vi "Solid Dilution Control-5.vi"() -> ()   [LabVIEW 2009]
uses:
  <vilib>/Instr/_visa.llb/VISA Configure Serial Port (Instr).vi
  <vilib>/DAQmx/configure/timing.llb/DAQmx Timing (Sample Clock).vi
  <vilib>/DAQmx/create/channels.llb/DAQmx Create Channel (AI-Strain-Strain Gage).vi
  <vilib>/DAQmx/read.llb/DAQmx Read (Analog 1D DBL 1Chan NSamp).vi
  <vilib>/Analysis/NI_AALBase.lvlib
panel:
  out "Target = Soln Size?":bool=TRUE
  in  "Fill Target":dbl=900.0
  out "Hydration (g)":dbl
  in  "SIM MASS":dbl=900.0
  in  "real":bool=TRUE
  out "# of Rows Saved":i32
  out "DAQ Loop":i32=644
  out "SCB Loop":i32=51
  out "Save Loop":i32=66
  out "Main Loop":i32=645
  out "Event Loop":i32=36
  in  "Tab Control":enum32{"DISPLAY", "CONFIGURE", "Load Cell"}(tab)
  in  "Settings":T1={"ON Settings"={"Enable Dynamic Setpoint?"=TRUE, "Enable Dynamic Dispense Time?"=TRUE, "Enable Drain Rate Functions"=TRUE, "Dispense Sample Time (s)"=0.1, "Mass Average Samples"=20, "ON Timeout (sec)"=300.0, "1st Setpoint (% of Target)"=90.0, "2nd Setpoint (% of Target)"=95.0, "3rd Setpoint (% of Target)"=100.0, "Measure Dispense Delay (sec)"=10.0, "Minimum Spray Time (s)"=2.0}, "OFF Settings"={"Drain Sample Time (s)"=0.1, "Drain Rate Ave Size"=100, "Drain Rate Limits (± g/sec)"=100.0, "Level Slope Range (± g/sec)"=0.05, "OFF Timeout (sec)"=300.0, "Near SP Slope Level (± g/sec)"=0.005, "Near Setpoint Threshold (%)"=99.0}, "Overshoot Settings"={"Time Limit (s)"=30.0, "Container MAX (g)"=1500.0, "Max FILL Slope (+/- g/sec)"=100.0, "% Overshot to Enable (>)"=3.0}, "FILL Timeout (s)"=300.0, "Full \nSettle Time (s)"=30.0, "Pre-Hydrate \nSpray Time (s)"=10.0, "Pre-Hydrate \nWait Time (s)"=30.0} {"OFF Settings"."Near SP Slope Level (± g/sec)" format="%.3g"; "OFF Settings"."Level Slope Range (± g/sec)" format="%.3g"}
  out "Values":T2 {"Drain Time (s)" format="%.2f"; "Drain Rate (g/sec)" format="%.2f"; "Spray Mass Loss (g)" format="%.2f"; "Time Elapsed (s)" format="%.2f"; "Time Target (s)" format="%.2f"; "Dynamic Setpoint (g)" format="%.2f"; "Static Setpoint (g)" format="%.2f"; "Grams to Setpoint" format="%.2f"; "Adjusted Mass (g)" format="%.2f"; "Dispense Rate (g/sec)" format="%.2f"; "Fill Mass (g)" format="%.2f"; "Fill Rate (g/sec)" format="%.2f"}
  in  "Tare":bool
  in  "Settings Button":bool
  in  "START Dispense":bool
  in  "STOP Dispense":bool
  in  "Fill Setpoint (g)":dbl
  in  "Dispense Setpoint (%)":dbl=10.0
  out "Mass Chart":T3(graph)={"Grams (SCB)"=0.0, "Fill Target"=900.0, "Dispense Target"=0.0}
  out "Signals":T4={"Dispense"=FALSE, "Fill"=FALSE, "Spray"=FALSE, "Drain"=TRUE, "Complete"=FALSE, "Fill Error"=FALSE, "Dispense Error"=FALSE, "Fill Timeout"=FALSE, "Dispense Timeout"=FALSE}
  in  "Overshoot Adjust?":bool
  out "Dispense Mode":T5(ring)
  out "Product Mass (g)":dbl format="%.2f"
  in  "Solution Size (g)":dbl=1000.0
  in  "Save Interval (s)":dbl=1.0
  in  "Write/Read Wait (ms)":u32=100
  in  "Event Loop Wait (ms)":i32=5000
  in  "File Path Input":path
  out "SCB Error":errorcluster={"status"=TRUE, "code"=-1073807343, "source"="Property Node (arg 1) in Read SCB via ESP (SubVI).vi->Solid Dilution Control-5.vi"}
  out "SCB Output":T6
  in  "SCB COM Port":refnum<visa-resource-name>="COM5"
  in  "SCB Baud Rate":u32=9600
  in  "DAQ COM Port":refnum<visa-resource-name>="COM4"
  in  "DAQ Baud Rate":u32=115200
  in  "Minimum Wait (ms)":u32=100
  in  "Module Address":i32=1
  in  "Relay Control":T7
  out "DAQ Com Error":errorcluster={"status"=TRUE, "code"=-1073807343, "source"="Property Node (arg 1) in VISA Configure Serial Port (Instr).vi->Solid Dilution Control-5.vi"}
  out "DAQ Error":errorcluster={"status"=TRUE, "code"=-1073807343, "source"="VISA Write in 7067 Relay Module (SubVI).vi->Solid Dilution Control-5.vi"}
  out "Relays Active?":bool
  out "SCB Com Error":errorcluster={"status"=TRUE, "code"=-1073807343, "source"="Property Node (arg 1) in VISA Configure Serial Port (Instr).vi->Solid Dilution Control-5.vi"}
  out "Save Error":errorcluster caption="Error Output"
  out "Weight (Grams)":dbl format="%.2f"
  out "Product Values":T8
  out "Spray Count":i32
  out "CDAQ Array":dbl[](graph)
  out "Grams (Tedea 1040 CDAQ)":dbl[](graph)
  in  "Minimum Value":dbl=-0.001 format="%0.3f"
  in  "Maximum Value":dbl=0.001 format="%0.3f"
  in  "CDAQ Channel":tag="Dev2/ai1"
  out "CDAQ Error":errorcluster={"status"=TRUE, "code"=-200220, "source"="DAQmx Create Channel (AI-Strain-Strain Gage).vi:1<append>\n<B>Device Specified: </B>Dev2\n\n<B>Task Name: </B>_unnamedTask<4>"}
  out "Raw Ave (Tedea 1040 CDAQ)":dbl=nan
  in  "Y LO (g)":dbl
  in  "Y HI (g)":dbl=5000.0
  in  "Set HI":bool
  in  "Set LO":bool
  out "CDAQ Sample Size":i32
  in  "CDAQ Wait (ms)":u32=100
  in  "CDAQ RATE":dbl=1000.0 caption="Rate" format="%0.2f"
  out "CDAQ Loop":i32
  in  "LO":dbl
  in  "HI":dbl
  in  "Save (Enable/Signal)":bool
  in  "STOP PROGRAM":bool
  # "SOLID DILUTION CONTROL SYSTEM"
  # "Program Last Updated 7/13/2010"
  # "SAVE\nENABLE"
  # "Blake Otting - Systems Engineering Lab - 2009 /2010"
  # "DISPENSE CONTROL"
  # "ONLY ADJUST\nBOLD VALUES!"
  # "GRAMS"
  # "SIGNAL"
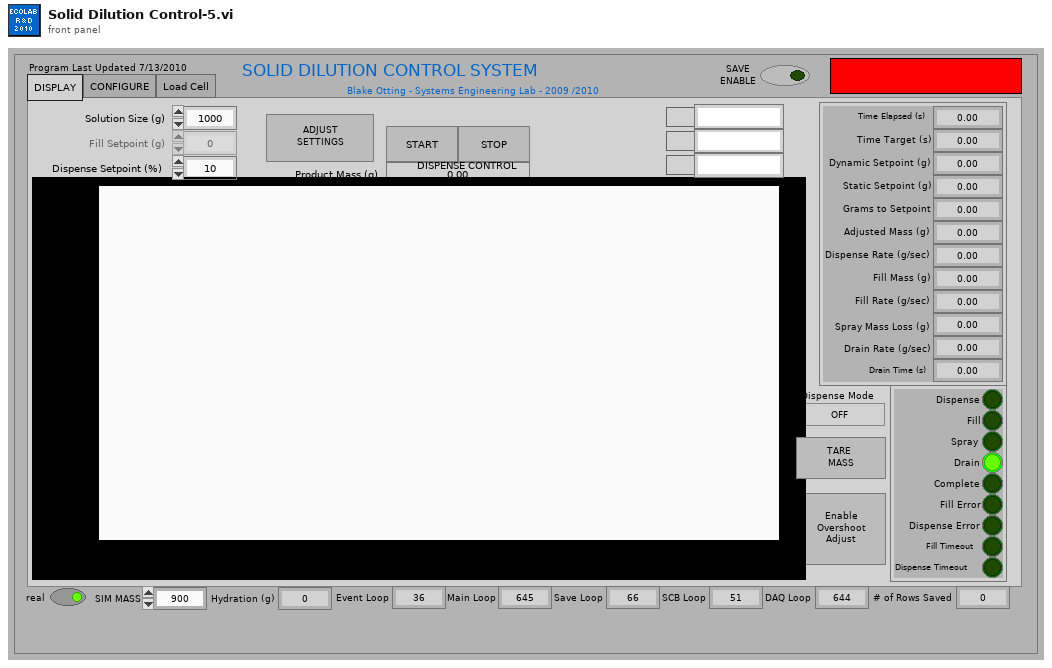
[diagram p1: front panel]
types:
  T1 = cluster{"ON Settings":cluster{"Enable Dynamic Setpoint?":bool, "Enable Dynamic Dispense Time?":bool, "Enable Drain Rate Functions":bool, "Dispense Sample Time (s)":dbl, "Mass Average Samples":i32, "ON Timeout (sec)":dbl, "1st Setpoint (% of Target)":dbl, "2nd Setpoint (% of Target)":dbl, "3rd Setpoint (% of Target)":dbl, "Measure Dispense Delay (sec)":dbl, "Minimum Spray Time (s)":dbl}, "OFF Settings":cluster{"Drain Sample Time (s)":dbl, "Drain Rate Ave Size":i32, "Drain Rate Limits (± g/sec)":dbl, "Level Slope Range (± g/sec)":dbl, "OFF Timeout (sec)":dbl, "Near SP Slope Level (± g/sec)":dbl, "Near Setpoint Threshold (%)":dbl}, "Overshoot Settings":cluster{"Time Limit (s)":dbl, "Container MAX (g)":dbl, "Max FILL Slope (+/- g/sec)":dbl, "% Overshot to Enable (>)":dbl}, "FILL Timeout (s)":dbl, "Full \nSettle Time (s)":dbl, "Pre-Hydrate \nSpray Time (s)":dbl, "Pre-Hydrate \nWait Time (s)":dbl}
  T2 = cluster{"Time Elapsed (s)":dbl, "Time Target (s)":dbl, "Dynamic Setpoint (g)":dbl, "Static Setpoint (g)":dbl, "Grams to Setpoint":dbl, "Adjusted Mass (g)":dbl, "Dispense Rate (g/sec)":dbl, "Fill Mass (g)":dbl, "Fill Rate (g/sec)":dbl, "Spray Mass Loss (g)":dbl, "Drain Rate (g/sec)":dbl, "Drain Time (s)":dbl}
  T3 = cluster{"Grams (SCB)":dbl, "Fill Target":dbl, "Dispense Target":dbl}
  T4 = cluster{"Dispense":bool, "Fill":bool, "Spray":bool, "Drain":bool, "Complete":bool, "Fill Error":bool, "Dispense Error":bool, "Fill Timeout":bool, "Dispense Timeout":bool}
  T5 = enum16{"OFF", "INITIAL", "FILL", "DISPENSE", "ADJUST"}
  T6 = cluster{"Sequence #":string, "Weight":string, "Status":string, "CRC & EOT":string}
  T7 = cluster{"Master (All Relays)":bool, "Relay1":bool, "Relay2":bool, "Relay3":bool, "Relay4":bool, "Relay5":bool, "Relay6":bool, "Relay7":bool}
  T8 = cluster{"Drain Delta":dbl, "Spray Delta":dbl, "Dispense Delta":dbl}
  T9 = enum8{"Enabled", "Disabled", "Disabled and Grayed Out"}
  T10 = cluster{"Grams (SCB)":dbl, "Fill Target":dbl, "Dispense Target":dbl}[]
  T11 = cluster{"Row Limit":i32, "Default File Name":string, "New File Daily?":bool, "Manual Save Interval?":bool}
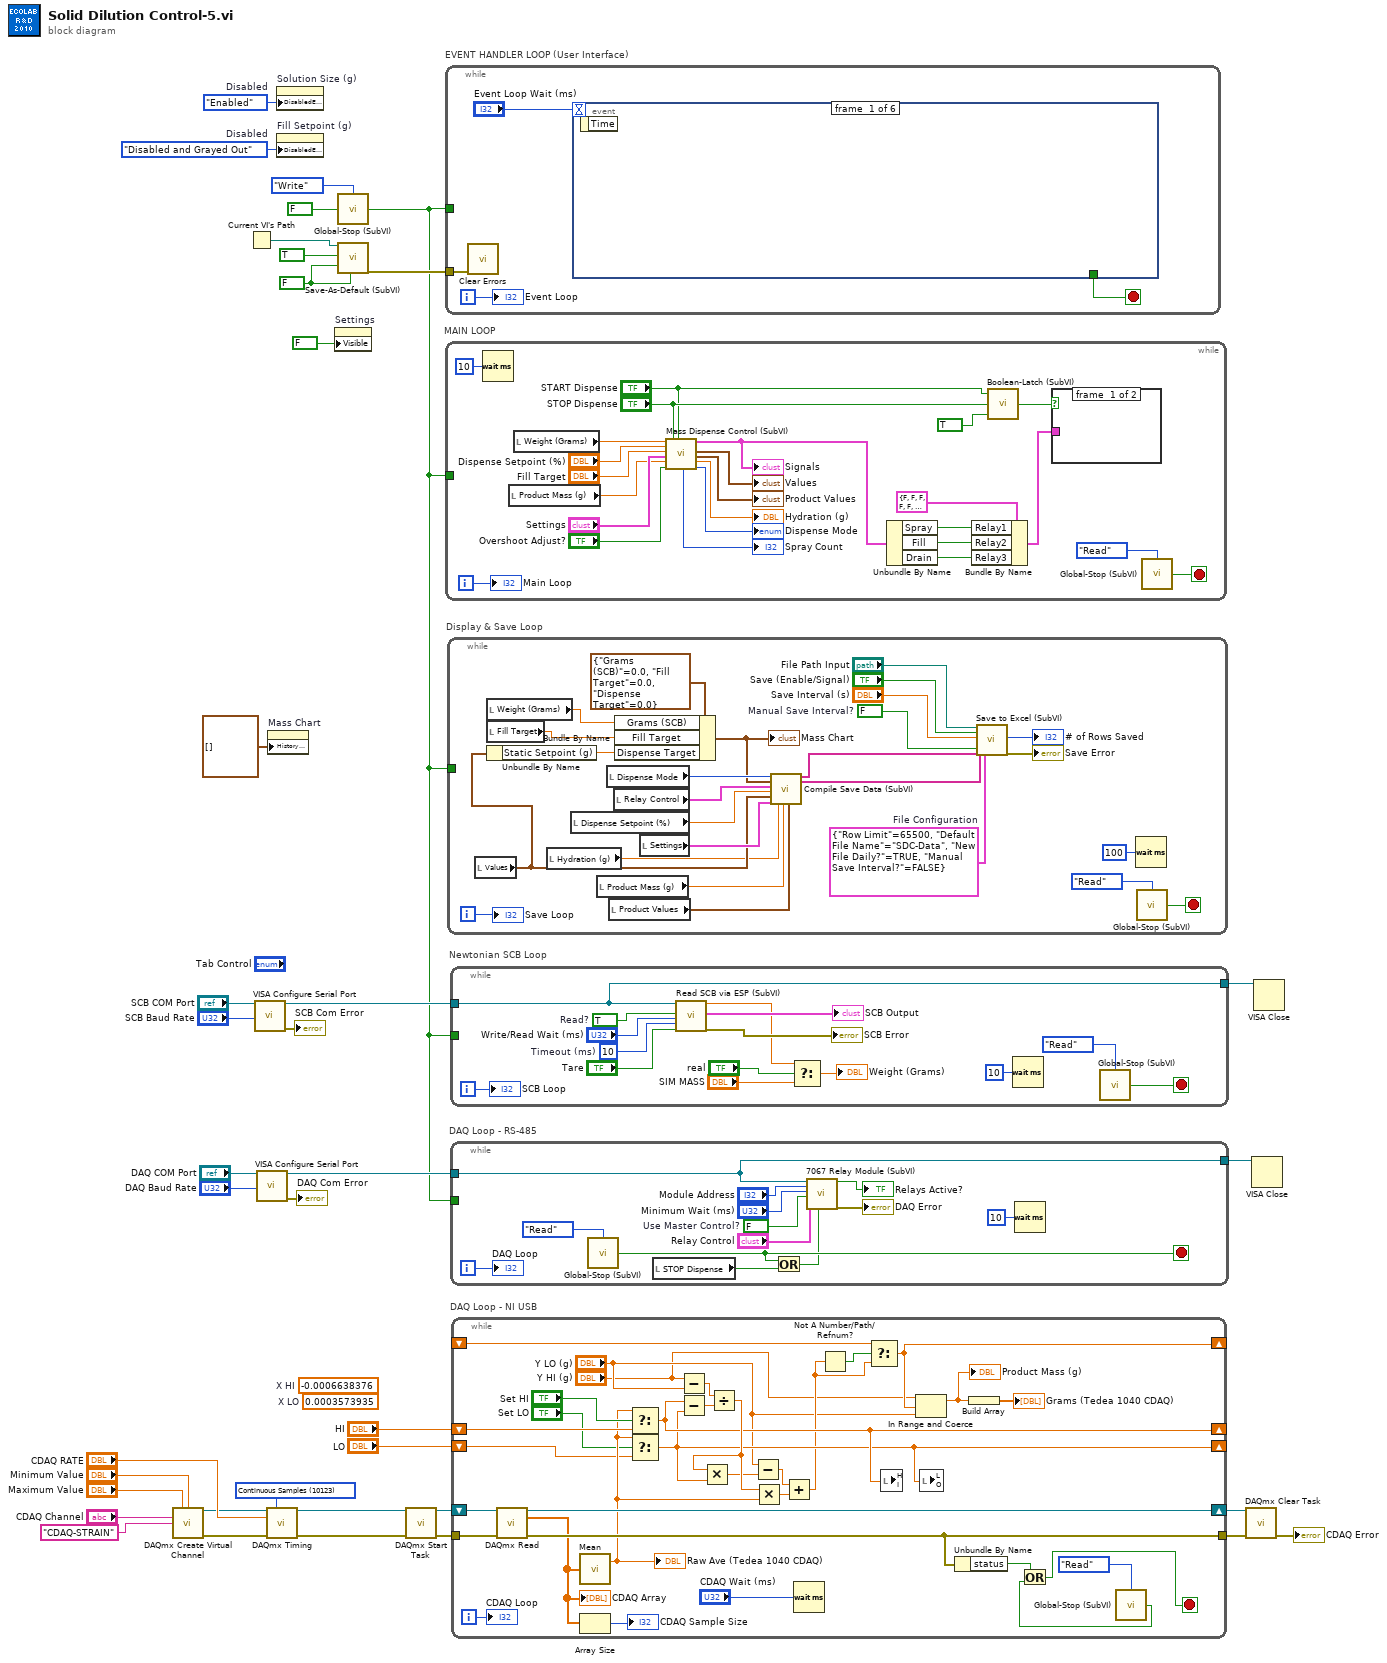
[diagram p0: block diagram]
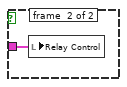
[diagram p2: hidden frame]
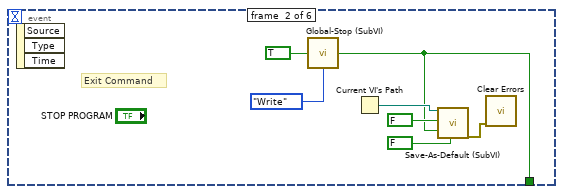
[diagram p3: hidden frame]
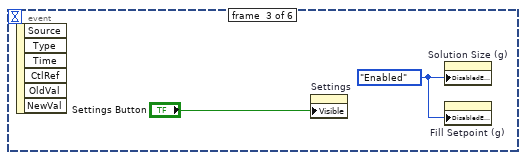
[diagram p4: hidden frame]
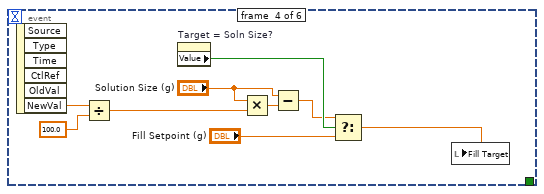
[diagram p5: hidden frame]
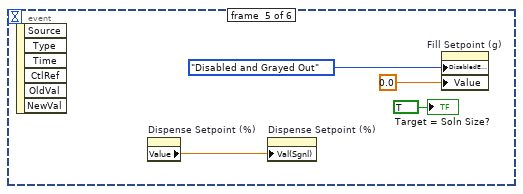
[diagram p6: hidden frame]
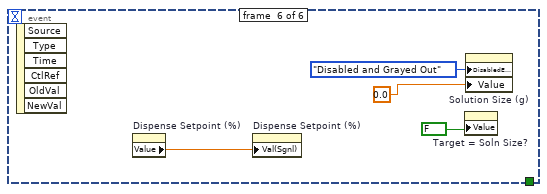
[diagram p7: hidden frame]
diagram:
  w1 = T9."Disabled and Grayed Out"  # Disabled
  w2 = T9."Enabled"  # Disabled
  (unwired) 0.0003573935  # X LO
  (unwired) -0.0006638376  # X HI
  w19 = 10123 items=["Finite Samples"=10178, "Continuous Samples"=10123] ("sample mode")
  w24 = FALSE ("Save Settings")
  n1 = call-poly <vilib>:"DAQmx Create Virtual Channel.vi"("maximum value"="Maximum Value", "minimum value"="Minimum Value", "physical channels"="CDAQ Channel", "name to assign"="CDAQ-STRAIN") -> ("task out"=w16:refnum<k21>, "error out"=w17:errorcluster)  [unwired: 8 in, 2 out]
  n2 = Current VI's Path() -> (path=w26:path)
  n3 = call-poly "VISA Configure Serial Port"("VISA resource name"="SCB COM Port", "baud rate (9600)"="SCB Baud Rate") -> ("VISA resource name out"=w31:refnum<visa-resource-name>, "error out"=→"SCB Com Error":errorcluster)  [unwired: 4 in, 8 out]
  n4 = call-poly "VISA Configure Serial Port"("VISA resource name"="DAQ COM Port", "baud rate (9600)"="DAQ Baud Rate") -> ("VISA resource name out"=w36:refnum<visa-resource-name>, "error out"=→"DAQ Com Error":errorcluster)  [unwired: 4 in, 8 out]
  n5 = call-poly <vilib>:"DAQmx Timing.vi"("task/channels in"=w16, "sample mode"=w19, "rate"="CDAQ RATE", "error in"=w17) -> ("task out"=w11:refnum<k21>, "error out"=w9:errorcluster)  [unwired: 3 in, 7 out]
  n6 = property on="Mass Chart" class="WFChart (strict)"("History Data"=T10 []) -> ()  [unwired: 2 in, 2 out]
  n7 = property on="Solution Size (g)" class="DigNum (strict)"("DisabledEnum"=w2) -> ()  [unwired: 2 in, 2 out]
  n8 = property on="Fill Setpoint (g)" class="DigNum (strict)"("DisabledEnum"=w1) -> ()  [unwired: 2 in, 2 out]
  n9 = property on="Settings" class="Clust (strict)"("Visible"=FALSE) -> ()  [unwired: 2 in, 2 out]
  n10 = call "Global-Stop (SubVI).vi"("Mode (Read)"=enum16{"Read", "Write"}."Write", "IN"=FALSE) -> ("OUT"=w20:bool)  [unwired: 2 out]
  n11 = call "Save-As-Default (SubVI).vi"("Current VI's Path"=w26, "Load Settings"=TRUE, "Save Settings"=w24, "Save and Exit"=w24) -> ("Save as Default Error"=w23:errorcluster)  [unwired: 15 in]
  n12 = call <vilib>:"DAQmx Start Task.vi"("task/channels in"=w11, "error in"=w9) -> ("task out"=w10:refnum<k21>, "error out"=w8:errorcluster)  [unwired: 12 out]
  n13 = while "EVENT HANDLER LOOP (User Interface)" {
    tunnel: w20 -> [_]
    tunnel: w23 -> [w40]
    i -> [w39]
    stop <- w42 stop-if-true
    n14 = call <vilib>:"Clear Errors.vi"("error in (no error)"=w40) -> ()  [unwired: 7 out]
    n15 = event shown="[3] \"Dispense Setpoint (%)\": Value Change" {
      selector: _ -> [_ _ _ _ _ _]
      dyn-events: _ -> [_ _ _ _ _ _]
      timeout: "Event Loop Wait (ms)" -> [_ _ _ _ _ _]
      tunnel: [_ w44 _ _ _ _] -> w42
      event #0 {
        n16 = event-data() -> ()  [unwired: 2 out]
      }
      event #1 {
        # "Exit Command"
        n17 = event-data() -> ()  [unwired: 4 out]
        n18 = call "Global-Stop (SubVI).vi"("Mode (Read)"=enum16{"Read", "Write"}."Write", "IN"=TRUE) -> ("OUT"=w44:bool)  [unwired: 2 out]
        n19 = Current VI's Path() -> (path=w46:path)
        n20 = call "Save-As-Default (SubVI).vi"("Current VI's Path"=w46, "Load Settings"=FALSE, "Save Settings"=w44, "Save and Exit"=FALSE ("Save Settings")) -> ("Save as Default Error"=w43:errorcluster)  [unwired: 15 in]
        n21 = call <vilib>:"Clear Errors.vi"("error in (no error)"=w43) -> ()  [unwired: 7 out]
      }
      event #2 {
        w50 = T9."Enabled" ("Disabled")
        n22 = event-data() -> ()  [unwired: 7 out]
        n23 = property on="Settings" class="Clust (strict)"("Visible"="Settings Button") -> ()  [unwired: 2 in, 2 out]
        n24 = property on="Solution Size (g)" class="DigNum (strict)"("DisabledEnum"=w50) -> ()  [unwired: 2 in, 2 out]
        n25 = property on="Fill Setpoint (g)" class="DigNum (strict)"("DisabledEnum"=w50) -> ()  [unwired: 2 in, 2 out]
      }
      event #3 {
        n26 = event-data() -> ("NewVal"=w59:dbl)  [unwired: 6 out]
        n27 = Divide(x=w59, y=100.0) -> (x/y=w56:dbl)
        n28 = property on="Target = Soln Size?" class="Bool (strict)"() -> ("Value"=w57:bool)  [unwired: 2 in, 2 out]
        n29 = Multiply(x="Solution Size (g)", y=w56) -> (x*y=w54:dbl)
        n30 = Subtract(x="Solution Size (g)", y=w54) -> (x-y=w53:dbl)
        n31 = Select(t=w53, s=w57, f="Fill Setpoint (g)") -> (s? t:f=w52:dbl)
        n32 = local write "Fill Target"(w52) -> ()
      }
      event #4 {
        n33 = event-data() -> ()  [unwired: 7 out]
        n34 = property on="Dispense Setpoint (%)" class="DigNum (strict)"() -> ("Value"=w61:dbl)  [unwired: 2 in, 2 out]
        n35 = property on="Dispense Setpoint (%)" class="DigNum (strict)"("Val(Sgnl)"=w61) -> ()  [unwired: 2 in, 2 out]
        n36 = property on="Fill Setpoint (g)" class="DigNum (strict)"("DisabledEnum"=T9."Disabled and Grayed Out" ("Disabled"), "Value"=0.0 ("Fill Setpoint (g)")) -> ()  [unwired: 2 in, 2 out]
        "Target = Soln Size?" <- TRUE
      }
      event #5 {
        n37 = event-data() -> ()  [unwired: 7 out]
        n38 = property on="Dispense Setpoint (%)" class="DigNum (strict)"() -> ("Value"=w65:dbl)  [unwired: 2 in, 2 out]
        n39 = property on="Dispense Setpoint (%)" class="DigNum (strict)"("Val(Sgnl)"=w65) -> ()  [unwired: 2 in, 2 out]
        n40 = property on="Target = Soln Size?" class="Bool (strict)"("Value"=FALSE) -> ()  [unwired: 2 in, 2 out]
        n41 = property on="Solution Size (g)" class="DigNum (strict)"("DisabledEnum"=T9."Disabled and Grayed Out" ("Disabled"), "Value"=0.0 ("Fill Setpoint (g)")) -> ()  [unwired: 2 in, 2 out]
      }
    }
    "Event Loop" <- w39
  }
  n42 = while "MAIN LOOP" {
    tunnel: w20 -> [_]
    i -> [w86]
    stop <- w89 stop-if-true
    n43 = Wait (ms)(milliseconds to wait=u32 10) -> ()  [unwired: 1 out]
    n44 = local read "Product Mass (g)"() -> (w73:dbl)
    n45 = local read "Weight (Grams)"() -> (w77:dbl)
    n46 = call "Mass Dispense Control (SubVI).vi"("Weight (Grams)"=w77, "Dispense Setpoint (%)"="Dispense Setpoint (%)", "Fill Setpoint (g)"="Fill Target", "Settings"="Settings", "Product Weight (g)"=w73, "Overshoot Adjust?"="Overshoot Adjust?", "STOP Dispense"="STOP Dispense", "START Dispense"="START Dispense") -> ("Spray Count"=→"Spray Count":i32, "Signals"=w78:T4, "Values"=→"Values":T2, "Product Values"=→"Product Values":T8, "Hydration (g)"=→"Hydration (g)":dbl, "Dispense Mode"=→"Dispense Mode":T5)  [unwired: 6 out]
    "Signals" <- w78
    n47 = Unbundle By Name(w78) -> ("Spray"=w85:bool, "Fill"=w84:bool, "Drain"=w90:bool)
    n48 = Bundle By Name(cluster=T7 {"Master (All Relays)"=FALSE, "Relay1"=FALSE, "Relay2"=FALSE, "Relay3"=FALSE, "Relay4"=FALSE, "Relay5"=FALSE, "Relay6"=FALSE, "Relay7"=FALSE} ("Relay Control"), "Relay1"=w85, "Relay2"=w84, "Relay3"=w90) -> (w87:T7)
    n49 = call "Boolean-Latch (SubVI).vi"("Reset on First Call (T)"=TRUE, "Reset"="STOP Dispense", "Trigger (Input)"="START Dispense") -> ("Latched? (Output)"=w88:bool)
    n50 = case shown="True" w88 {
      tunnel: w87 -> [_ w94]
      frame #0 {
      }
      frame #1 {
        n51 = local write "Relay Control"(w94) -> ()
      }
    }
    n52 = call "Global-Stop (SubVI).vi"("Mode (Read)"=enum16{"Read", "Write"}."Read") -> ("OUT"=w89:bool)  [unwired: 1 in, 2 out]
    "Main Loop" <- w86
  }
  n53 = while "Display & Save Loop" {
    tunnel: w20 -> [_]
    i -> [w111]
    stop <- w118 stop-if-true
    w97 = T11 {"Row Limit"=65500, "Default File Name"="SDC-Data", "New File Daily?"=TRUE, "Manual Save Interval?"=FALSE}  # File Configuration
    w113 = FALSE  # Manual Save Interval?
    n54 = local read "Values"() -> (w102:T2)
    n55 = local read "Weight (Grams)"() -> (w104:dbl)
    n56 = local read "Fill Target"() -> (w95:dbl)
    n57 = Unbundle By Name(w102) -> ("Static Setpoint (g)"=w109:dbl)
    n58 = local read "Hydration (g)"() -> (w98:dbl)
    n59 = local read "Dispense Setpoint (%)"() -> (w106:dbl)
    n60 = local read "Product Mass (g)"() -> (w100:dbl)
    n61 = local read "Dispense Mode"() -> (w103:T5)
    n62 = local read "Product Values"() -> (w99:T8)
    n63 = local read "Relay Control"() -> (w107:T7)
    n64 = Bundle By Name(cluster=T3 {"Grams (SCB)"=0.0, "Fill Target"=0.0, "Dispense Target"=0.0} ("Conductivity"), "Grams (SCB)"=w104, "Fill Target"=w95, "Dispense Target"=w109) -> (w101:T3)
    "Mass Chart" <- w101
    n65 = local read "Settings"() -> (w105:T1)
    n66 = call "Compile Save Data (SubVI).vi"("Dispense Mode"=w103, "Mass Chart"=w101, "Relay Control"=w107, "Dispense Setpoint (%)"=w106, "Values"=w102, "Settings"=w105, "Hydration (g)"=w98, "Product Mass (g)"=w100, "Product Values"=w99) -> ("Data Array Output"=w96:string[], "Column Header Text Array"=w108:string[])  [unwired: 9 out]
    n67 = call "Save to Excel (SubVI).vi"("File Path Input"="File Path Input", "Save (Enable/Signal)"="Save (Enable/Signal)", "Save Interval (s)"="Save Interval (s)", "Column Header Array"=w108, "Data Array (Row)"=w96, "File Configuration"=w97, "Change Save Location?"=w113) -> ("# of Rows Saved"=→"# of Rows Saved":i32, "Error Output"=→"Save Error":errorcluster)  [unwired: 8 in, 3 out]
    n68 = Wait (ms)(milliseconds to wait=u32 100) -> ()  [unwired: 1 out]
    n69 = call "Global-Stop (SubVI).vi"("Mode (Read)"=enum16{"Read", "Write"}."Read") -> ("OUT"=w118:bool)  [unwired: 1 in, 2 out]
    "Save Loop" <- w111
  }
  n70 = while "Newtonian SCB Loop" {
    tunnel: w31 -> [w127]
    tunnel: [w127] -> w28
    tunnel: w20 -> [_]
    i -> [w125]
    stop <- w129 stop-if-true
    w135 = TRUE  # Read?
    w133 = u32 10  # Timeout (ms)
    n71 = call "Read SCB via ESP (SubVI).vi"("COM Port Input"=w127, "Manual Write Command"=w135, "Write/Read Wait (ms)"="Write/Read Wait (ms)", "Timeout (ms)"=w133, "Tare"="Tare") -> ("Weight (Grams)"=w123:dbl, "SCB Output"=→"SCB Output":T6, "Error Output"=→"SCB Error":errorcluster)  [unwired: 12 out]
    n72 = Select(t=w123, s="real", f="SIM MASS") -> (s? t:f=→"Weight (Grams)":dbl)
    n73 = Wait (ms)(milliseconds to wait=u32 10) -> ()  [unwired: 1 out]
    n74 = call "Global-Stop (SubVI).vi"("Mode (Read)"=enum16{"Read", "Write"}."Read") -> ("OUT"=w129:bool)  [unwired: 1 in, 2 out]
    "SCB Loop" <- w125
  }
  n75 = while "DAQ Loop - RS-485" {
    tunnel: w36 -> [w140]
    tunnel: [w140] -> w27
    tunnel: w20 -> [_]
    i -> [w139]
    stop <- w137 stop-if-true
    w146 = FALSE  # Use Master Control?
    n76 = call "Global-Stop (SubVI).vi"("Mode (Read)"=enum16{"Read", "Write"}."Read") -> ("OUT"=w137:bool)  [unwired: 1 in, 2 out]
    n77 = local read "STOP Dispense"() -> (w138:bool)
    n78 = Or(x=w137, y=w138) -> (x .or. y?=w136:bool)
    n79 = call "7067 Relay Module (SubVI).vi"("COM Port"=w140, "Module Address"="Module Address", "Minimum Wait (ms)"="Minimum Wait (ms)", "Use Master Control?"=w146, "Relay Control"="Relay Control", "E-STOP (ALL OFF)"=w136) -> ("Relays Active?"=→"Relays Active?":bool, "Error Output"=→"DAQ Error":errorcluster)  [unwired: 12 out]
    n80 = Wait (ms)(milliseconds to wait=u32 10) -> ()  [unwired: 1 out]
    "DAQ Loop" <- w139
  }
  n81 = while "DAQ Loop - NI USB" {
    tunnel: w8 -> [w168]
    tunnel: [w167] -> w7
    shift-right: [w164] -> w5
    shift-left: w10 -> [w169]
    shift-right: [w157] -> _
    shift-left: "HI" -> [w162]
    shift-right: [w156] -> _
    shift-left: "LO" -> [w159]
    shift-right: [w151] -> _
    shift-left: _ -> [w154]
    i -> [w158]
    stop <- w170 stop-if-true
    n82 = call-poly <vilib>:"DAQmx Read.vi"("task/channels in"=w169, "error in"=w168) -> ("task out"=w164:refnum<k21>, "data"=w165:dbl[], "error out"=w167:errorcluster)  [unwired: 1 in, 10 out]
    "CDAQ Array" <- w165
    n83 = call <vilib>:"Mean.vi"("X"=w165) -> ("mean"=w161:dbl)  [unwired: 1 out]
    "Raw Ave (Tedea 1040 CDAQ)" <- w161
    n84 = Array Size(array=w165) -> (size(s)=→"CDAQ Sample Size":i32)
    n85 = Select(t=w161, s="Set HI", f=w162) -> (s? t:f=w157:dbl)
    n86 = Select(t=w161, s="Set LO", f=w159) -> (s? t:f=w156:dbl)
    n87 = Subtract(x="Y HI (g)", y="Y LO (g)") -> (x-y=w173:dbl)
    n88 = Subtract(x=w157, y=w156) -> (x-y=w174:dbl)
    n89 = Divide(x=w173, y=w174) -> (x/y=w176:dbl)
    n90 = Multiply(x=w176, y=w156) -> (x*y=w175:dbl)
    n91 = Subtract(x="Y LO (g)", y=w175) -> (x-y=w177:dbl)
    n92 = Multiply(x=w176, y=w161) -> (x*y=w178:dbl)
    n93 = Add(x=w177, y=w178) -> (x+y=w153:dbl)
    n94 = Wait (ms)(milliseconds to wait="CDAQ Wait (ms)") -> ()  [unwired: 1 out]
    n95 = Not A Number/Path/Refnum?(number/path/refnum=w153) -> (NaN/Path/Refnum?=w155:bool)
    n96 = Select(t=w154, s=w155, f=w153) -> (s? t:f=w151:dbl)
    n97 = local write "HI"(w157) -> ()
    n98 = In Range and Coerce(upper limit="Y HI (g)", x=w151, lower limit="Y LO (g)") -> (coerced(x)=w149:dbl)  [unwired: 1 out]
    "Product Mass (g)" <- w149
    n99 = local write "LO"(w156) -> ()
    n100 = Unbundle By Name(w167) -> ("status"=w172:bool)
    n101 = Build Array(w149) -> (→"Grams (Tedea 1040 CDAQ)":dbl[])
    n102 = call "Global-Stop (SubVI).vi"("Mode (Read)"=enum16{"Read", "Write"}."Read") -> ("OUT"=w171:bool)  [unwired: 1 in, 2 out]
    n103 = Or(x=w172, y=w171) -> (x .or. y?=w170:bool)
    "CDAQ Loop" <- w158
  }
  n104 = call <vilib>:"DAQmx Clear Task.vi"("task in"=w5, "error in"=w7) -> ("error out"=→"CDAQ Error":errorcluster)  [unwired: 13 out]
  n105 = VISA Close(VISA resource name=w27) -> ()  [unwired: 1 in, 1 out]
  n106 = VISA Close(VISA resource name=w28) -> ()  [unwired: 1 in, 1 out]
